vi "DisableEnableControlVolt (SubVI).vi"(10 "enabled":bool, 11 "Menu in":refnum<k9>) -> ()   [LabVIEW 2017]
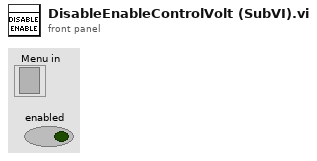
[diagram p1: front panel]
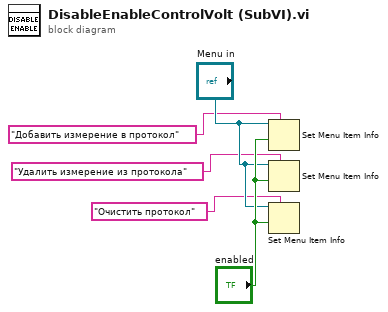
[diagram p0: block diagram]
diagram:
  n1 = Set Menu Item Info(7:"Добавить измерение в протокол" ("item name"), 9:"enabled", 11:"Menu in") -> ()  [unwired: 4 in, 2 out]
  n2 = Set Menu Item Info(7:"Удалить измерение из протокола" ("item name"), 9:"enabled", 11:"Menu in") -> ()  [unwired: 4 in, 2 out]
  n3 = Set Menu Item Info(7:"Очистить протокол" ("item name"), 9:"enabled", 11:"Menu in") -> ()  [unwired: 4 in, 2 out]
